vi "CSTK_MCListbox_Designer_UpdateColHdrsOtherAttr.vi"(7 "引用输入":T1, 8 "错误输入（无错误）":errorcluster, 11 "MCListbox引用句柄":refnum<vi>) -> (0 "错误输出":errorcluster)   [LabVIEW 2015, in "CSTK_MCListbox Designer.lvlib"]
uses:
  CSTK_MCListbox Designer.lvlib
  _CSTK_MCListbox_Designer_RowAttr.ctl
  <vilib>/Utility/miscctls.llb/LVRowAndColumnTypeDef.ctl
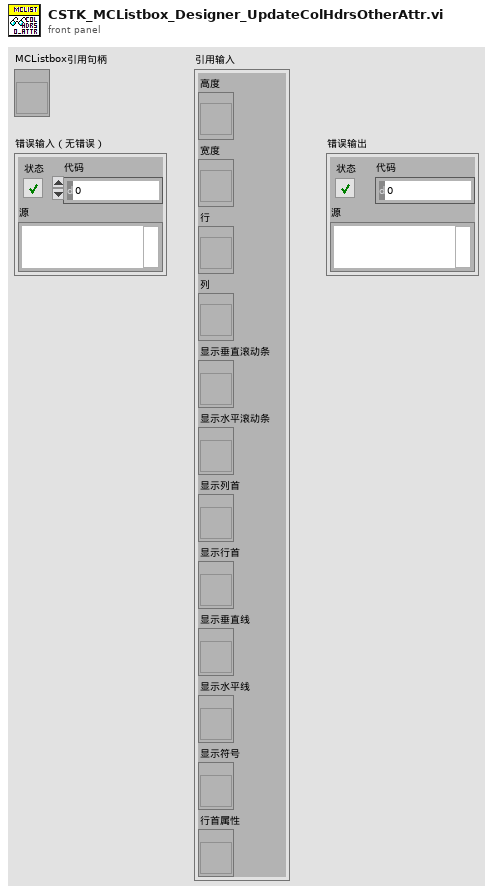
[diagram p1: front panel]
types:
  T1 = cluster{"高度":refnum<vi>, "宽度":refnum<vi>, "行":refnum<vi>, "列":refnum<vi>, "显示垂直滚动条":refnum<vi>, "显示水平滚动条":refnum<vi>, "显示列首":refnum<vi>, "显示行首":refnum<vi>, "显示垂直线":refnum<vi>, "显示水平线":refnum<vi>, "显示符号":refnum<vi>, "行首属性":refnum<vi>}
  T2 = typedef "CSTK_MCListbox Designer.lvlib/_CSTK_MCListbox_Designer_RowAttr.ctl" = cluster{"宽度":u32, "粗体":bool, "斜体":bool, "对齐":enum16{"Left", "Center", "Right"}}
  T3 = typedef "LVRowAndColumnTypeDef.ctl" = cluster{"Row":i32, "Column":i32}
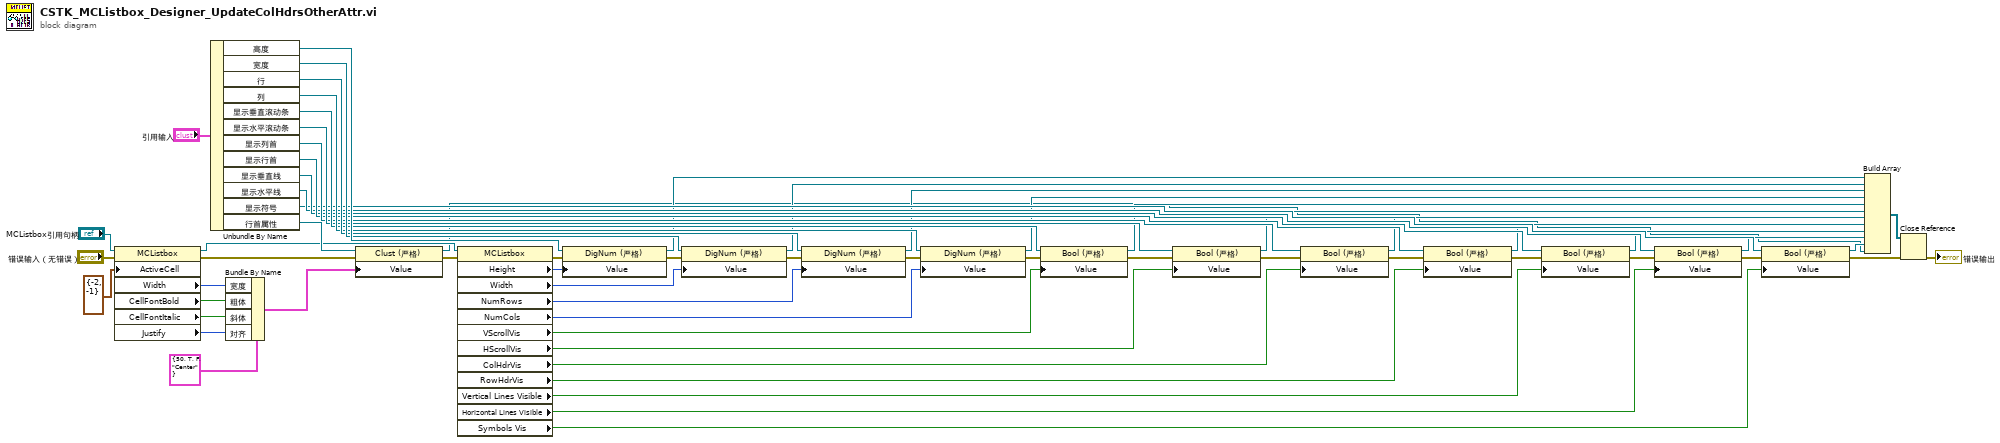
[diagram p0: block diagram]
diagram:
  n1 = property class="MCListbox"(reference="MCListbox引用句柄", error in="错误输入（无错误）", "ActiveCell"=T3 {"Row"=-2, "Column"=-1} ("活动单元格:活动单元格")) -> (reference out=w5:refnum<vi>, error out=w7:errorcluster, "Width"=w10:u32, "CellFontBold"=w8:bool, "CellFontItalic"=w1:bool, "Justify"=w9:enum16{"Left", "Center", "Right"})
  n2 = Unbundle By Name("引用输入") -> ("高度"=w59:refnum<vi>, "宽度"=w57:refnum<vi>, "行"=w53:refnum<vi>, "列"=w50:refnum<vi>, "显示垂直滚动条"=w48:refnum<vi>, "显示水平滚动条"=w46:refnum<vi>, "显示列首"=w41:refnum<vi>, "显示行首"=w40:refnum<vi>, "显示垂直线"=w35:refnum<vi>, "显示水平线"=w34:refnum<vi>, "显示符号"=w31:refnum<vi>, "行首属性"=w13:refnum<vi>)
  n3 = Bundle By Name(cluster=T2 {"宽度"=50, "粗体"=TRUE, "斜体"=FALSE, "对齐"=enum."Center"} ("值"), "宽度"=w10, "粗体"=w8, "斜体"=w1, "对齐"=w9) -> (w11:T2)
  n4 = property on="属性节点" class="Clust (严格)"(reference=w13, error in=w7, "Value"=w11) -> (reference out=w2:refnum<vi>, error out=w3:errorcluster)
  n5 = property class="MCListbox"(reference=w5, error in=w3) -> (error out=w62:errorcluster, "Height"=w58:u32, "Width"=w56:u32, "NumRows"=w52:u32, "NumCols"=w49:u32, "VScrollVis"=w47:bool, "HScrollVis"=w43:bool, "ColHdrVis"=w39:bool, "RowHdrVis"=w38:bool, "Vertical Lines Visible"=w33:bool, "Horizontal Lines Visible"=w32:bool, "Symbols Vis"=w30:bool)  [unwired: 1 out]
  n6 = property on="属性节点" class="DigNum (严格)"(reference=w59, error in=w62, "Value"=w58) -> (reference out=w27:refnum<vi>, error out=w55:errorcluster)
  n7 = property on="属性节点" class="DigNum (严格)"(reference=w57, error in=w55, "Value"=w56) -> (reference out=w26:refnum<vi>, error out=w54:errorcluster)
  n8 = property on="属性节点" class="DigNum (严格)"(reference=w53, error in=w54, "Value"=w52) -> (reference out=w25:refnum<vi>, error out=w51:errorcluster)
  n9 = property on="属性节点" class="DigNum (严格)"(reference=w50, error in=w51, "Value"=w49) -> (reference out=w24:refnum<vi>, error out=w45:errorcluster)
  n10 = property on="属性节点" class="Bool (严格)"(reference=w48, error in=w45, "Value"=w47) -> (reference out=w23:refnum<vi>, error out=w44:errorcluster)
  n11 = property on="属性节点" class="Bool (严格)"(reference=w46, error in=w44, "Value"=w43) -> (reference out=w22:refnum<vi>, error out=w28:errorcluster)
  n12 = property on="属性节点" class="Bool (严格)"(reference=w41, error in=w28, "Value"=w39) -> (reference out=w21:refnum<vi>, error out=w42:errorcluster)
  n13 = property on="属性节点" class="Bool (严格)"(reference=w40, error in=w42, "Value"=w38) -> (reference out=w20:refnum<vi>, error out=w36:errorcluster)
  n14 = property on="属性节点" class="Bool (严格)"(reference=w35, error in=w36, "Value"=w33) -> (reference out=w19:refnum<vi>, error out=w37:errorcluster)
  n15 = property on="属性节点" class="Bool (严格)"(reference=w34, error in=w37, "Value"=w32) -> (reference out=w18:refnum<vi>, error out=w29:errorcluster)
  n16 = property on="属性节点" class="Bool (严格)"(reference=w31, error in=w29, "Value"=w30) -> (reference out=w17:refnum<vi>, error out=w15:errorcluster)
  n17 = Build Array(w27, w26, w25, w24, w23, w22, w21, w20, w19, w18, w17, w2) -> (w16:refnum<vi>[])
  n18 = Close Reference(reference=w16, error in (no error)=w15) -> (error out=→"错误输出":errorcluster)
